vi "Global.vi"() -> ()   [LabVIEW 2011]
uses:
  event.ctl
panel:
  out "events":refnum<queue>
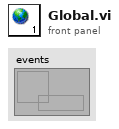
[diagram p1: front panel]
diagram:
